vi "Write Element of Curr Position.vi"(8 "error in (no error)":errorcluster, 9 "Position idx":i32, 10 "Wheel":i32, 11 "Filter Wheel in":refnum<class "Filter Wheel.lvclass">) -> (0 "error out":errorcluster, 3 "Filter Wheel out":refnum<class "Filter Wheel.lvclass">)   [LabVIEW 2024, in "Filter Wheel.lvclass"]
uses:
  Filter Wheel.lvclass
  Filter Wheel.lvclass/Filter Wheel.ctl
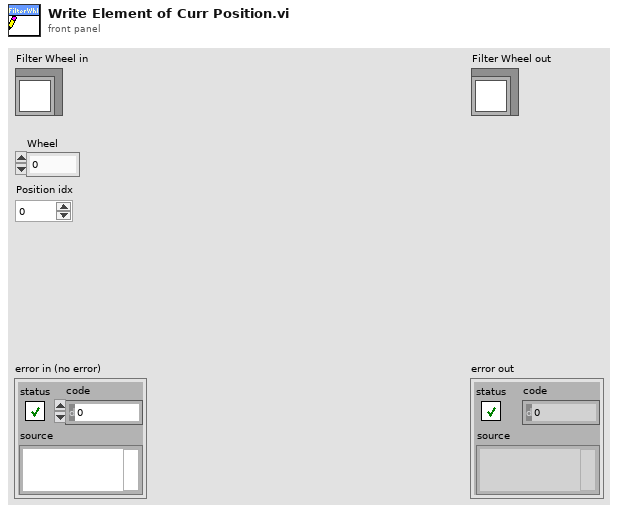
[diagram p1: front panel]
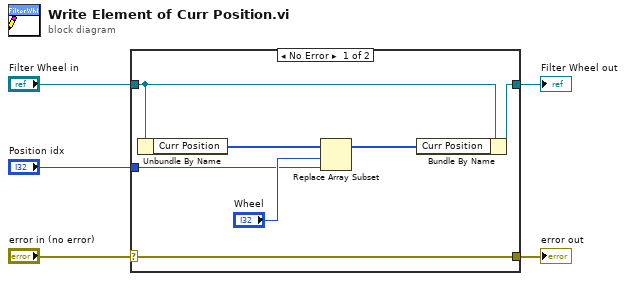
[diagram p0: block diagram]
diagram:
  n1 = case shown="No Error" "error in (no error)" {
    selector: "error in (no error)" -> [w12 w13]
    tunnel: [w12 w13] -> w4
    tunnel: [w11 w14] -> w2
    tunnel: "Filter Wheel in" -> [w10 w14]
    tunnel: "Position idx" -> [w6 _]
    frame No Error {
      n2 = Unbundle By Name(w10) -> ("Curr Position"=w9:i32[])
      n3 = Replace Array Subset(array=w9, new element=w6, index="Wheel") -> (w8:i32[])
      n4 = Bundle By Name(cluster=w10, "Curr Position"=w8) -> (w11:refnum<class "Filter Wheel.lvclass">)
    }
    frame Error {
    }
  }
  "error out" <- w4
  "Filter Wheel out" <- w2
